vi "Signals to JSON.vi"(11 "Signal Sessions":T1) -> (3 "JSON string":string)   [LabVIEW 2021]
uses:
  863f65c0-6e08-4c3b-92ae-c38da8f40fe4.vi
  controls/JSON sigs.ctl
panel:
  out "error out":errorcluster
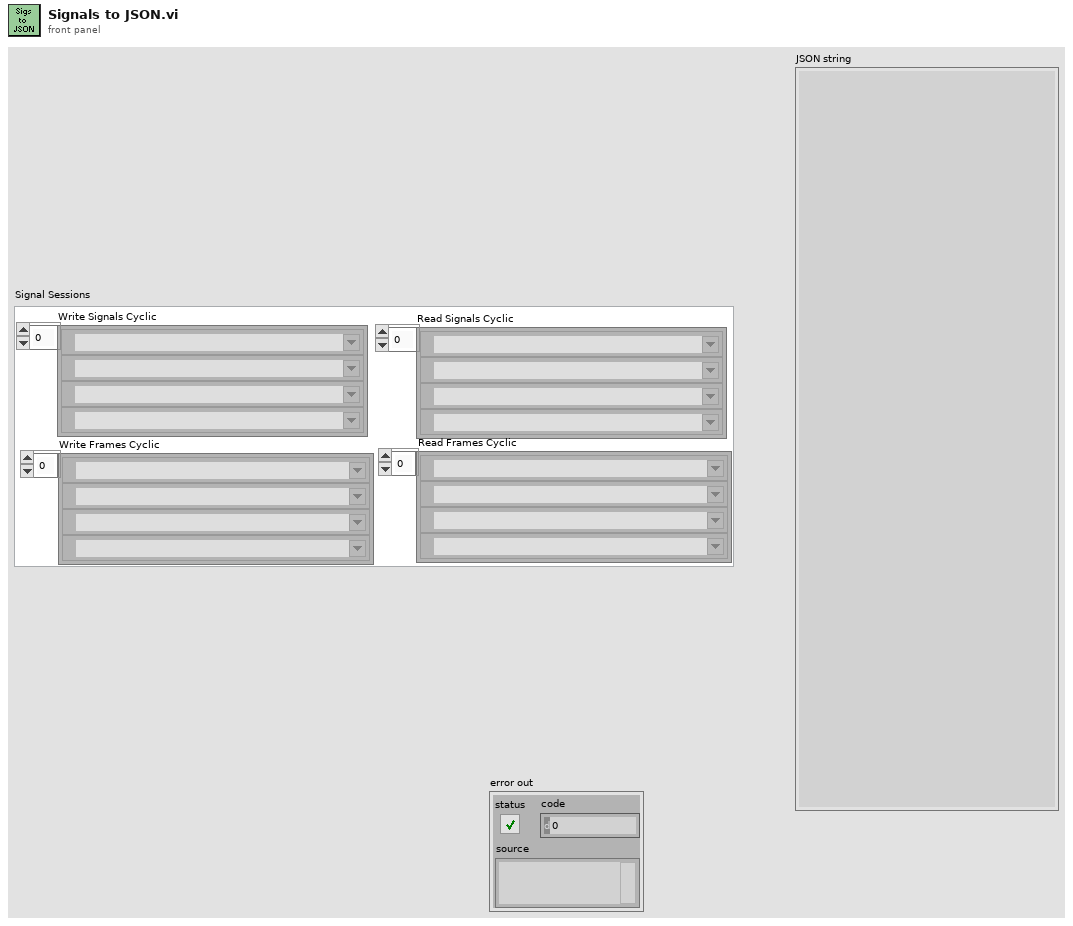
[diagram p1: front panel]
types:
  T1 = typedef "JSON sigs.ctl" = cluster{"Read Signals Cyclic":refnum<k21>[], "Write Signals Cyclic":refnum<k21>[], "Write Frames Cyclic":refnum<k21>[], "Read Frames Cyclic":refnum<k21>[]}
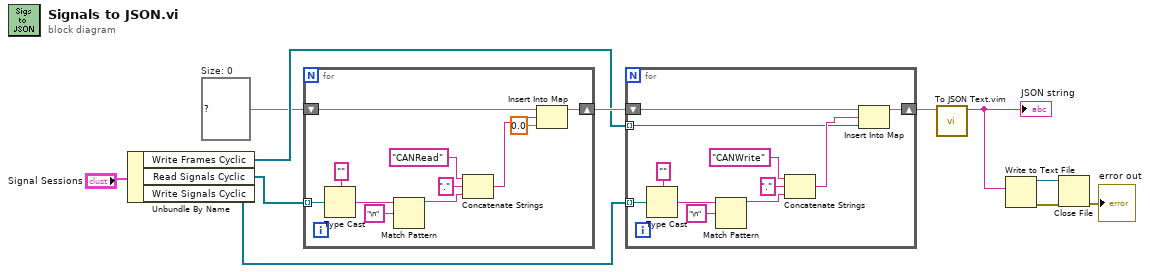
[diagram p0: block diagram]
diagram:
  w1 = map{string, dbl} {}  # Size: 0
  n1 = Unbundle By Name("Signal Sessions") -> ("Write Frames Cyclic"=w6:refnum<k21>[], "Read Signals Cyclic"=w11:refnum<k21>[], "Write Signals Cyclic"=w9:refnum<k21>[])
  n2 = for {
    tunnel: w11 -> [w21] mode=indexing
    shift-right: [w14] -> w8
    shift-left: w1 -> [w13]
    n3 = Type Cast(type="", x=w21) -> (*(type *) &x=w18:string)
    n4 = Match Pattern(string=w18, regular expression="\n") -> (before substring=w16:string)  [unwired: 1 in, 3 out]
    n5 = Concatenate Strings("CANRead" ("type"), "." ("string"), w16) -> (w15:string)
    n6 = Insert Into Map(map in=w13, key=w15, value=0.0) -> (map out=w14:map{string, dbl})  [unwired: 2 out]
  }
  n7 = for {
    tunnel: w9 -> [w32] mode=indexing
    shift-right: [w25] -> w7
    shift-left: w8 -> [w24]
    tunnel: w6 -> [w23] mode=indexing
    n8 = Type Cast(type="", x=w32) -> (*(type *) &x=w29:string)
    n9 = Match Pattern(string=w29, regular expression="\n") -> (before substring=w27:string)  [unwired: 1 in, 3 out]
    n10 = Concatenate Strings("CANWrite" ("type"), "." ("string"), w27) -> (w26:string)
    n11 = Insert Into Map(map in=w24, key=w26, value=w23) -> (map out=w25:map{string, dbl})  [unwired: 2 out]
  }
  n12 = call "To JSON Text.vim"("Anything"=w7) -> ("<JSON>"=w5:string)  [unwired: 9 in, 1 out]
  "JSON string" <- w5
  n13 = Write to Text File(text=w5) -> (refnum out=w3:refnum<file>, error out=w4:errorcluster)  [unwired: 3 in, 1 out]
  n14 = Close File(refnum=w3, error in=w4) -> (error out=→"error out":errorcluster)  [unwired: 1 out]
